vi "Range Converter.vi"(8 "error in (no error)":errorcluster, 11 "Max V/Div":dbl format="%#_13g") -> (0 "error out":errorcluster, 3 "Range":u32(ring)=6 items=["10 mV", "20 mV", "50 mV", "100 mV", "200 mV", "500 mV", "1 V", "2 V", "5 V", "10 V", "20 V", "50 V ", "100 V"])   [LabVIEW 2018, in "PicoScope 3000a.lvlib" / "PicoScope 3000a.lvclass"]
doc: "As the PicoScope 3000a only supports up to +/- 20 V, this VI check that the Max V/Div on each signals does not surpass the supported maximum. The logic of the VI is that if there is a worse case scenario of only 2 divisions retrieved, one for + and another for the - portion of a periodic signal, then the selected range will be capable of showing it.\nExample:\nTwo signals are feed to the Oscope, no offset"
uses:
  PicoScope 3000a.lvclass
panel:
  out "number":dbl
  out "Strings []":string[](array[string])
  in  "Max Range":u32(ring)=10 items=["10 mV", "20 mV", "50 mV", "100 mV", "200 mV", "500 mV", "1 V", "2 V", "5 V", "10 V", "20 V", "50 V ", "100 V"]
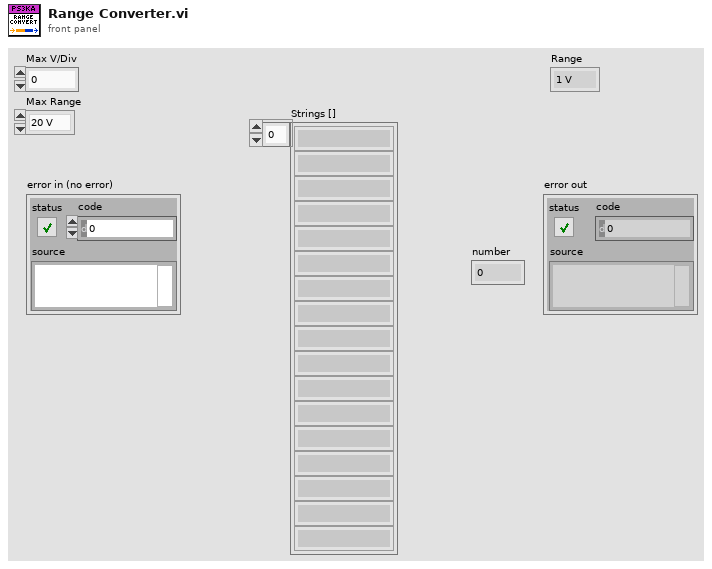
[diagram p1: front panel]
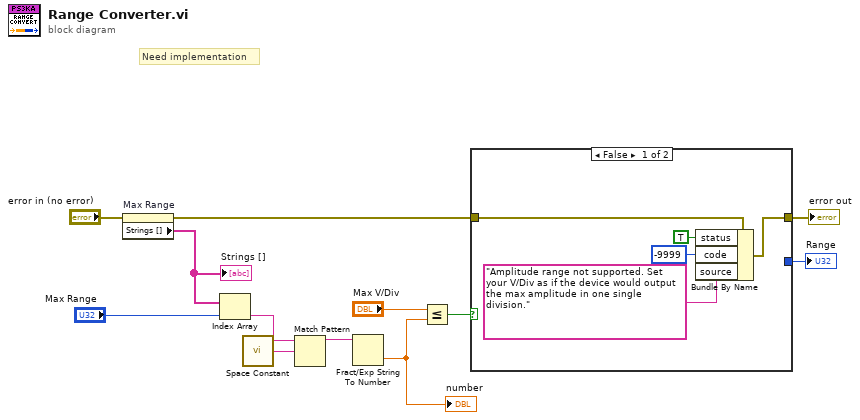
[diagram p0: block diagram]
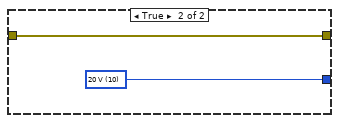
[diagram p2: hidden frame]
diagram:
  # "Need implementation"
  n1 = property on="Max Range" class="Ring (strict)"(error in="error in (no error)") -> (error out=w3:errorcluster, "Strings []"=w8:string[])  [unwired: 1 in, 1 out]
  "Strings []" <- w8
  n2 = Index Array(array=w8, index="Max Range") -> (element=w11:string)
  n3 = call <vilib>:"Space Constant.vi"() -> ("String"=w10:string)
  n4 = Match Pattern(string=w11, regular expression=w10) -> (before substring=w9:string)  [unwired: 1 in, 3 out]
  n5 = Fract/Exp String To Number(string=w9) -> (number=w5:dbl)  [unwired: 3 in, 1 out]
  "number" <- w5
  n6 = Less Or Equal?(x="Max V/Div", y=w5) -> (x <= y?=w4:bool)
  n7 = case shown="False" w4 {
    tunnel: w3 -> [w17 w18]
    tunnel: [_ w19] -> w2
    tunnel: [w16 w18] -> w1
    frame False {
      n8 = Bundle By Name(cluster=w17, "status"=TRUE, "code"=-9999, "source"="Amplitude range not supported. Set your V/Div as if the device would output the max amplitude in one single division.") -> (w16:errorcluster)
    }
    frame True {
      w19 = u32 10 items=["10 mV", "20 mV", "50 mV", "100 mV", "200 mV", "500 mV", "1 V", "2 V", "5 V", "10 V", "20 V", "50 V ", "100 V"] ("Range")
    }
  }
  "Range" <- w2
  "error out" <- w1
